vi "Read Data as Mono8 Image.vi"(8 "error in (no error)":errorcluster, 11 "Buffer in":refnum<class "Buffer.lvclass">) -> (0 "error out":errorcluster, 2 "Image":u8[][](array[numeric]), 3 "Buffer":refnum<class "Buffer.lvclass">)   [LabVIEW 2020, in "Buffer.lvclass"]
uses:
  Buffer.lvclass
  Buffer.lvclass/Buffer.ctl
  bin/gindustrialcam_32-1.dll
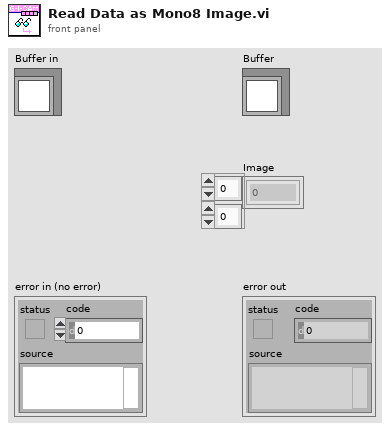
[diagram p1: front panel]
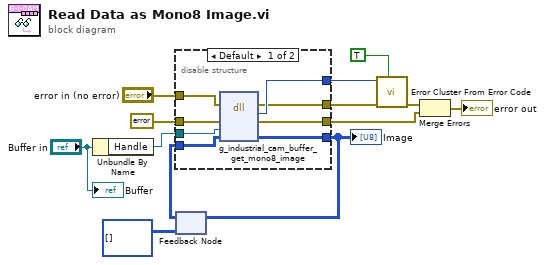
[diagram p0: block diagram]
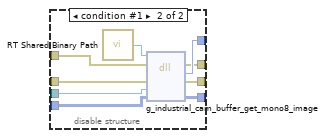
[diagram p2: hidden frame]
diagram:
  n1 = Unbundle By Name("Buffer in") -> ("Handle"=w1:refnum<data-value>)
  n2 = feedback #1(u8[][] [] ("Image")) -> (w3:u8[][])
  n3 = disable-structure shown="Default" {
    disable-tunnel: errorcluster {"status"=FALSE, "code"=0, "source"=""} ("error constant") -> [w21 w30]
    disable-tunnel: [w20 w29] -> w10
    disable-tunnel: [w19 w28] -> w8
    disable-tunnel: [w18 w27] -> w7
    disable-tunnel: "error in (no error)" -> [w17 w26]
    disable-tunnel: [w16 w25] -> w4
    disable-tunnel: w3 -> [w15 w24]
    disable-tunnel: w1 -> [w14 w23]
    frame condition #0 (active) {
      n4 = dll-call lib="C:/serenial/lib/g-industrial-camera/LabVIEW/g_industrial_cam/bin/gindustrialcam_*-1.*" fn="g_industrial_cam_buffer_get_mono8_image"(error in=w17, "err"=w21, "edvr"=w14, "Image"=w15) -> (error out=w18:errorcluster, "Mg_Error"=w19:i32, "err"=w20:errorcluster, "Image"=w16:u8[][])  [unwired: 3 in, 1 out]
    }
    frame condition #1 {
      n5 = call "RT Shared Binary Path.vi"() -> ("Path"=w22:path)
      n6 = dll-call lib="C:/serenial/lib/g-industrial-camera/LabVIEW/g_industrial_cam/bin/gindustrialcam_*-1.*" fn="g_industrial_cam_buffer_get_mono8_image"(path in=w22, error in=w26, "err"=w30, "edvr"=w23, "Image"=w24) -> (error out=w27:errorcluster, "Mg_Error"=w28:i32, "err"=w29:errorcluster, "Image"=w25:u8[][])  [unwired: 2 in, 1 out]
    }
  }
  "Image" <- w4
  n7 = feedback-in #1(w4) -> ()
  n8 = call <vilib>:"Error Cluster From Error Code.vi"("show call chain? (False)"=TRUE, "error in (no error)"=w7, "error code (0)"=w8) -> ("error out"=w9:errorcluster)  [unwired: 6 in]
  n9 = Merge Errors(w9, w10) -> (→"error out":errorcluster)
  "Buffer" <- "Buffer in"
